vi "24-type_digital_bis.vi"(3 "this":i32, 4 "button":i32, 5 "digital tmp in":bool=TRUE, 6 "settings in":T2={"Auto1"=TRUE, "Auto2"=TRUE, "Rel1"=TRUE, "Rel2"=TRUE, "Filt1"=TRUE, "Filt2"=TRUE, "Rate"=enum."Med", "Range1"=enum."10mV", "Range2"=enum."100mV", "Filt3"=TRUE, "Filt4"=TRUE, "Rel temp"=TRUE, "Analog1"=FALSE, "Analog2"=FALSE, "Analog temp"=FALSE, "Digital1"=TRUE, "Digital2"=TRUE, "Digital temp "=TRUE, "Window1"=enum."0,01%", "Window2"=enum."0,01%", "Window temp"=enum."0,01%", "RDGS1"="010", "RDGS2"="010", "RDGS temp"="010", "Type_type1"=TRUE, "Type_type2"=TRUE, "Type_type temp"=TRUE, "LSync"=FALSE, "Unit"=enum."C", "Sens"=TRUE, "Type tcoupl"=enum."J", "Junc"=TRUE, "prevState"=0}) -> (0 "next state":i32, 1 "digital tmp out":bool, 2 "settings out":T1)   [LabVIEW 2017]
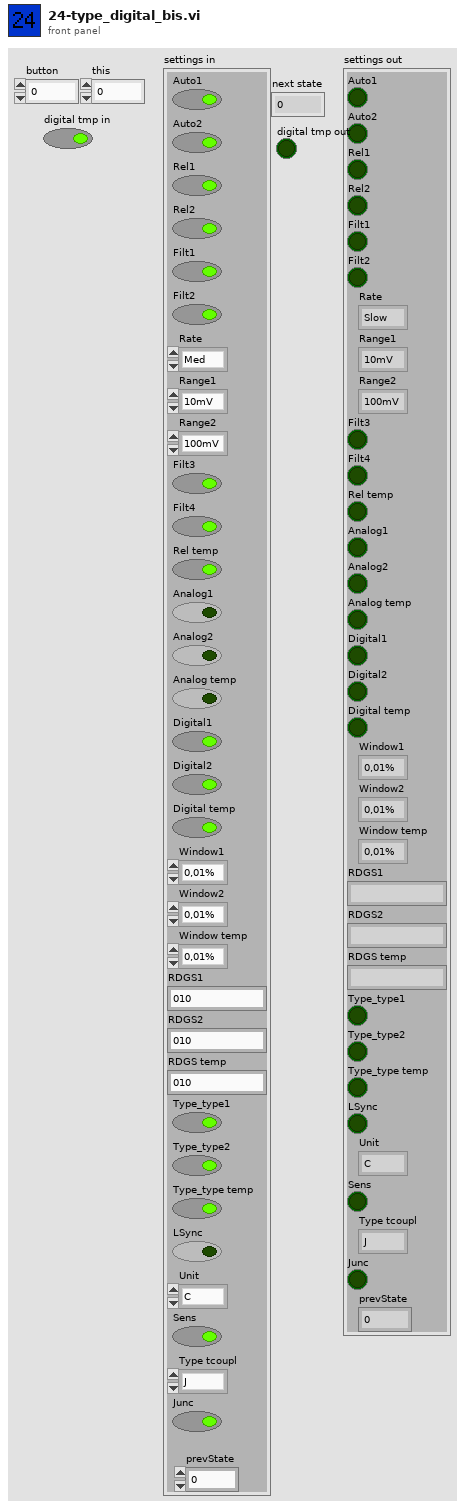
[diagram p1: front panel]
types:
  T1 = cluster{"Auto1":bool, "Auto2":bool, "Rel1":bool, "Rel2":bool, "Filt1":bool, "Filt2":bool, "Rate":enum16{"Slow", "Med", "Fast"}, "Range1":enum16{"10mV", "100mV", "1V", "10V", "100V"}, "Range2":enum16{"100mV", "1V", "10V"}, "Filt3":bool, "Filt4":bool, "Rel temp":bool, "Analog1":bool, "Analog2":bool, "Analog temp":bool, "Digital1":bool, "Digital2":bool, "Digital temp ":bool, "Window1":enum16{"0,01%", "0,1%", "1%", "10%", "None"}, "Window2":enum16{"0,01%", "0,1%", "1%", "10%", "None"}, "Window temp":enum16{"0,01%", "0,1%", "1%", "10%", "None"}, "RDGS1":string, "RDGS2":string, "RDGS temp":string, "Type_type1":bool, "Type_type2":bool, "Type_type temp":bool, "LSync":bool, "Unit":enum16{"C", "K", "F"}, "Sens":bool, "Type tcoupl":enum16{"J", "K", "T", "E", "R", "S", "B", "N"}, "Junc":bool, "prevState":dbl}
  T2 = cluster{"Auto1":bool, "Auto2":bool, "Rel1":bool, "Rel2":bool, "Filt1":bool, "Filt2":bool, "Rate":enum16{"Slow", "Med", "Fast"}, "Range1":enum16{"10mV", "100mV", "1V", "10V", "100V"}, "Range2":enum16{"100mV", "1V", "10V"}, "Filt3":bool, "Filt4":bool, "Rel temp":bool, "Analog1":bool, "Analog2":bool, "Analog temp":bool, "Digital1":bool, "Digital2":bool, "Digital temp ":bool, "Window1":enum16{"0,01%", "0,1%", "1%", "10%", "None"}, "Window2":enum16{"0,01%", "0,1%", "1%", "10%", "None"}, "Window temp":enum16{"0,01%", "0,1%", "1%", "10%", "None"}, "RDGS1":string, "RDGS2":string, "RDGS temp":string, "Type_type1":bool, "Type_type2":bool, "Type_type temp":bool, "LSync":bool, "Unit":enum16{"C", "K", "F"}, "Sens":bool, "Type tcoupl":enum16{"J", "K", "T", "E", "R", "S", "B", "N"}, "Junc":bool, "prevState":i32}
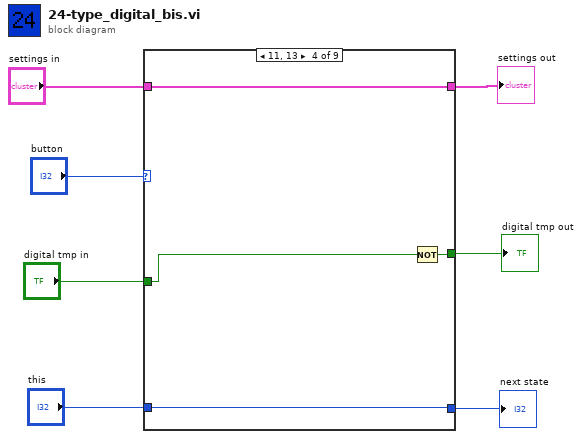
[diagram p0: block diagram]
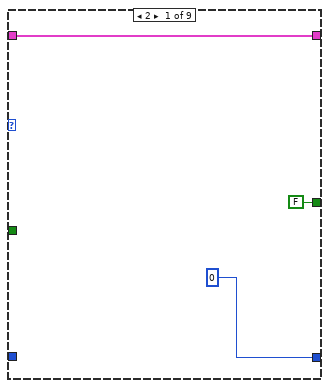
[diagram p2: hidden frame]
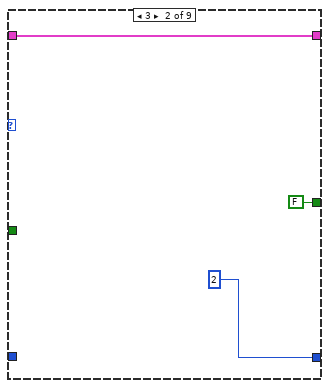
[diagram p3: hidden frame]
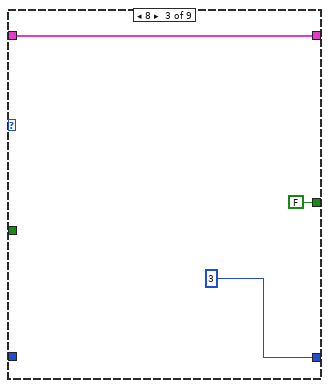
[diagram p4: hidden frame]
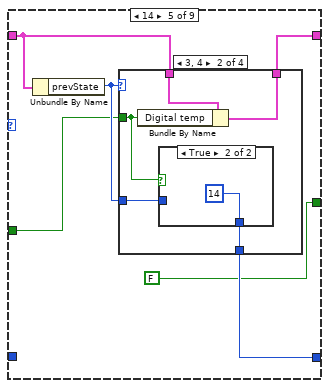
[diagram p5: hidden frame]
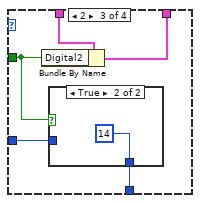
[diagram p8: hidden frame]
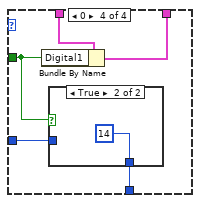
[diagram p10: hidden frame]
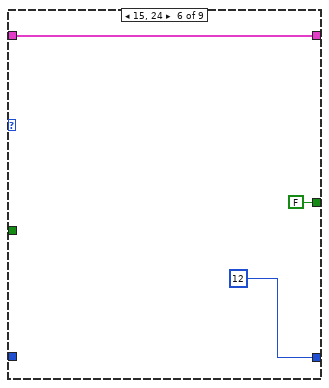
[diagram p12: hidden frame]
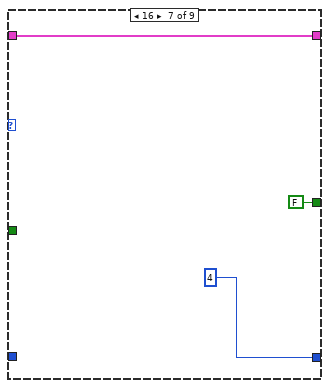
[diagram p13: hidden frame]
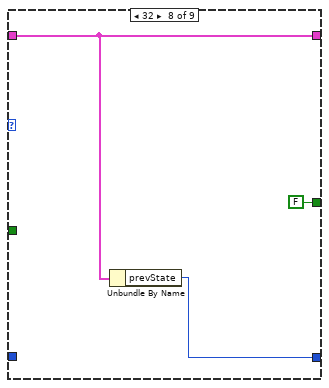
[diagram p14: hidden frame]
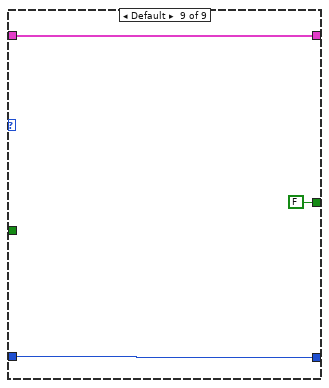
[diagram p15: hidden frame]
diagram:
  n1 = case shown="11, 13" "button" {
    tunnel: [0 ("this") 2 3 w17 w25 12 ("this") 4 w57 w60] -> w4
    tunnel: "this" -> [_ _ _ w17 _ _ _ _ w60]
    tunnel: "settings in" -> [w10 w12 w15 w20 w26 w52 w54 w58 w61]
    tunnel: [w10 w12 w15 w20 w23 w52 w54 w58 w61] -> w3
    tunnel: [FALSE FALSE FALSE w19 FALSE FALSE FALSE FALSE FALSE] -> w2
    tunnel: "digital tmp in" -> [_ _ _ w18 w22 _ _ _ _]
    frame 2 {
    }
    frame 3 {
    }
    frame 8 {
    }
    frame 11, 13 {
      n2 = Not(x=w18) -> (.not. x?=w19:bool)
    }
    frame 14 {
      n3 = Unbundle By Name(w26) -> ("prevState"=w24:i32)
      n4 = case shown="3, 4" w24 {
        tunnel: w26 -> [w27 w31 w38 w45]
        tunnel: [w28 w33 w40 w47] -> w25
        tunnel: w24 -> [w28 w32 w39 w46]
        tunnel: [w27 w30 w37 w44] -> w23
        tunnel: w22 -> [_ w29 w36 w43]
        frame Default {
        }
        frame 3, 4 {
          n5 = Bundle By Name(cluster=w31, "Digital temp"=w29) -> (w30:T2)
          n6 = case shown="True" w29 {
            tunnel: [w34 14] -> w33
            tunnel: w32 -> [w34 _]
            frame False {
            }
            frame True {
            }
          }
        }
        frame 2 {
          n7 = Bundle By Name(cluster=w38, "Digital2"=w36) -> (w37:T2)
          n8 = case shown="True" w36 {
            tunnel: [w41 14] -> w40
            tunnel: w39 -> [w41 _]
            frame False {
            }
            frame True {
            }
          }
        }
        frame 0 {
          n9 = Bundle By Name(cluster=w45, "Digital1"=w43) -> (w44:T2)
          n10 = case shown="True" w43 {
            tunnel: [w48 14] -> w47
            tunnel: w46 -> [w48 _]
            frame False {
            }
            frame True {
            }
          }
        }
      }
    }
    frame 15, 24 {
    }
    frame 16 {
    }
    frame 32 {
      n11 = Unbundle By Name(w58) -> ("prevState"=w57:i32)
    }
    frame Default {
    }
  }
  "next state" <- w4
  "settings out" <- w3
  "digital tmp out" <- w2
